vi "Peltier Temperature Test.vi"(8 "error in":errorcluster) -> (0 "error out":errorcluster)   [LabVIEW 2014]
uses:
  CAN Communication/Peltier/Typedefs/Peltier Temperature Sensors.ctl
  CAN Communication/Peltier/Peltier.lvclass
panel:
  in  "Stop":bool
  out "Timeout":i32
  in  "Values":i32(listbox)
  out "Error":errorcluster
  # "Peltier Temperature Test"
  # "This test performs functionality\ntesting on the Peltier Board.\n\nPlease standby while the test is\nin progress..."
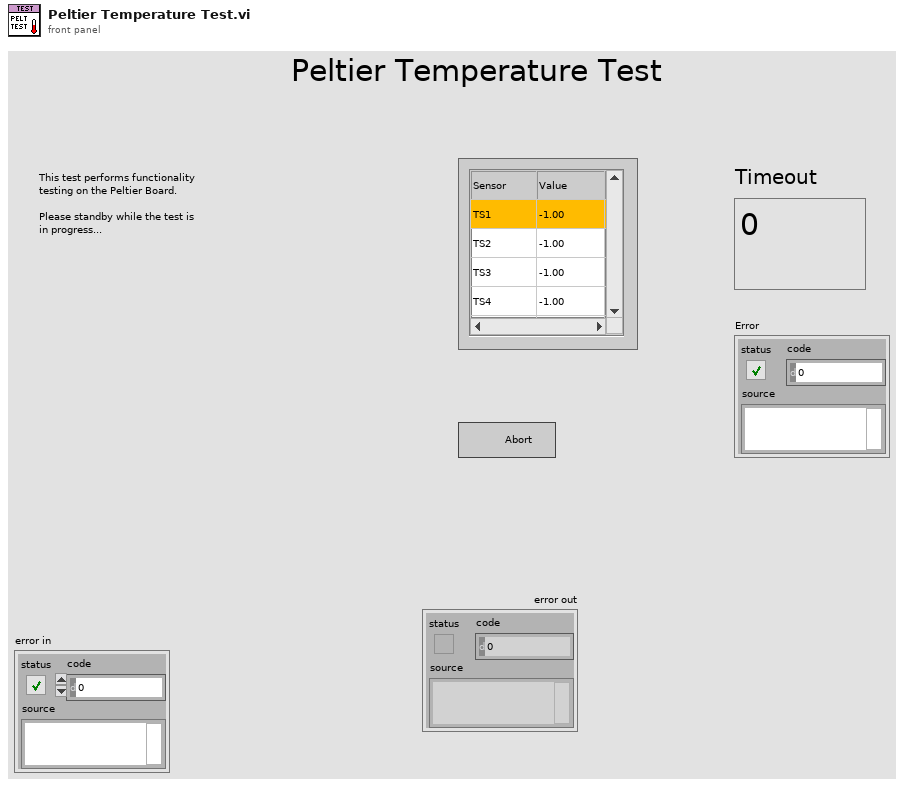
[diagram p1: front panel]
types:
  T1 = typedef "Peltier.lvclass/Peltier Temperature Sensors.ctl" = u16
  T2 = typedef "Peltier.lvclass/Session Handle.ctl" = refnum<data-value>
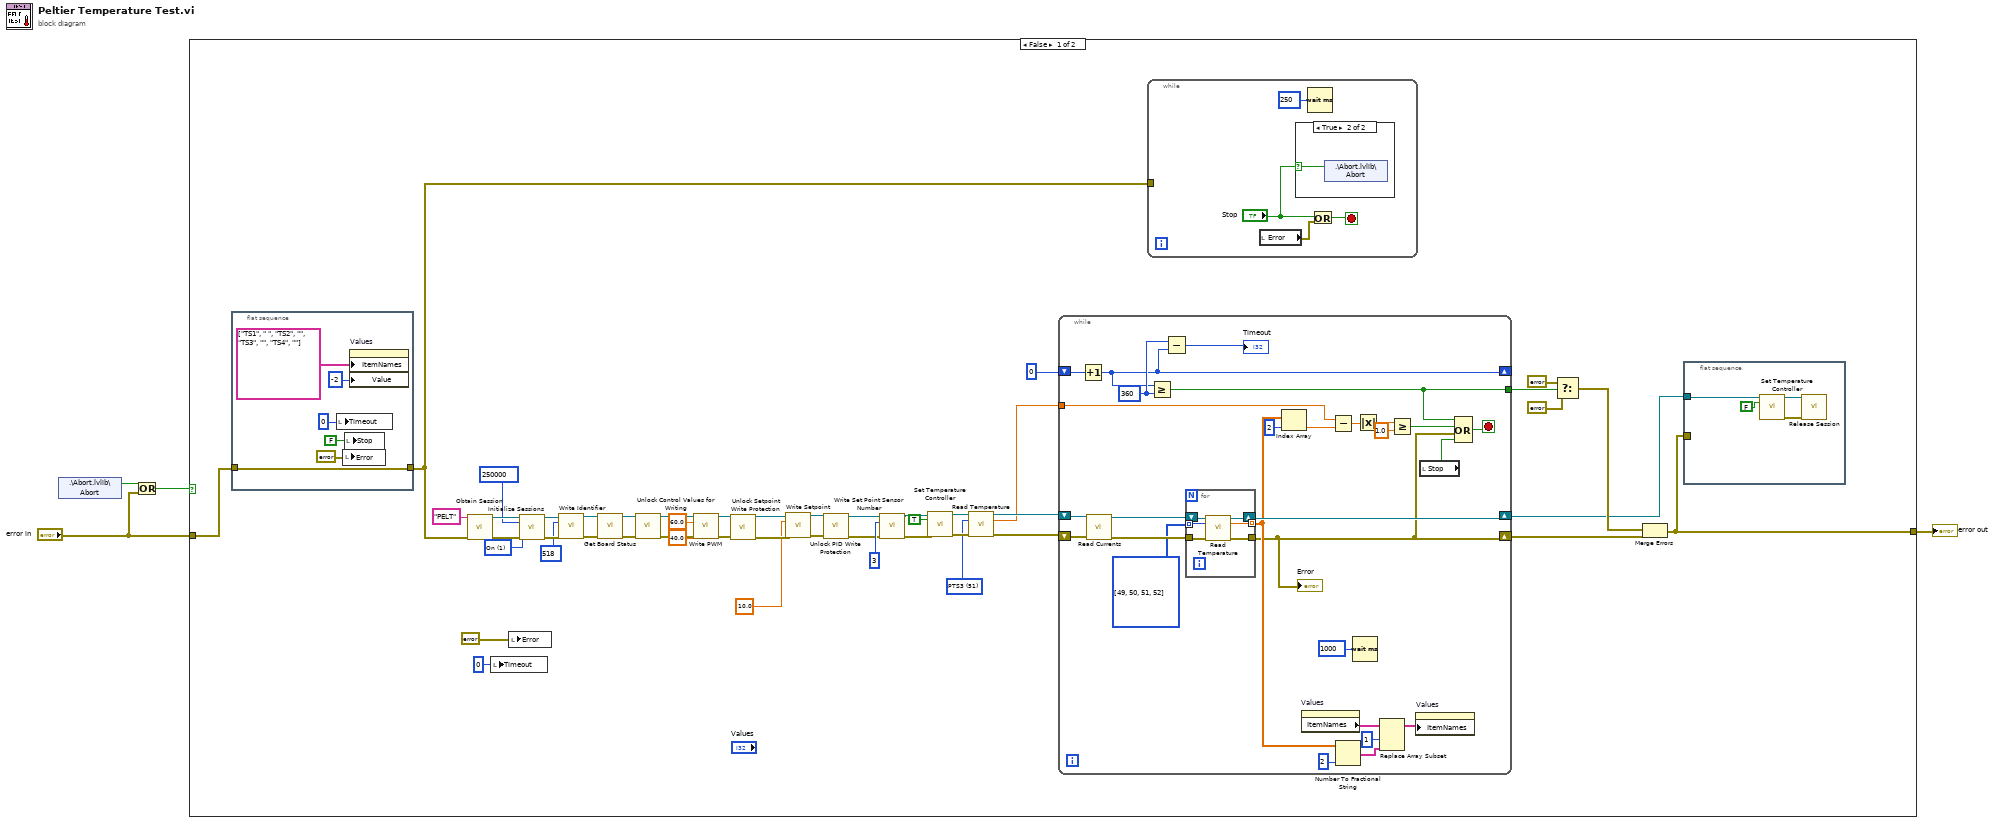
[diagram p0: block diagram]
diagram:
  n1 = shared-variable ".\\Abort.lvlib\\Abort"() -> (w3:bool)  [unwired: 1 in, 1 out]
  n2 = Or(x=w3, y="error in") -> (x .or. y?=w1:bool)
  n3 = case shown="False" w1 {
    tunnel: "error in" -> [w7 w101]
    tunnel: [w5 w101] -> w4
    frame False {
      w21 = T1 51 items=["PTS1"=49, "PTS2"=50, "PTS3"=51, "PTS4"=52, "PTS5"=53, "PTS6"=54] ("Pelt Temp Sensors")
      w47 = u32 1 items=["Off", "On"] ("Termination")
      n4 = flat-sequence {
        tunnel: w7 -> [w56]
        tunnel: [w56] -> w6
        frame #0 {
          n5 = local write "Timeout"(0 ("Timeout")) -> ()
          n6 = local write "Error"(errorcluster {"status"=FALSE, "code"=0, "source"=""} ("Error")) -> ()
          n7 = local write "Stop"(FALSE ("Stop")) -> ()
          n8 = property on="Values" class="MCListbox (strict)"("ItemNames"=string[][] [["TS1", " "], ["TS2", ""], ["TS3", ""], ["TS4", ""]] ("Item Names"), "Value"=-2 ("Values")) -> ()  [unwired: 2 in, 2 out]
        }
      }
      n9 = call "Obtain Session.vi"("Session  Name ()"="PELT", "error in (no error)"=w6) -> ("Session Handle"=w50:T2, "error out"=w49:errorcluster)  [unwired: 12 in]
      n10 = local write "Timeout"(0 ("Timeout")) -> ()
      n11 = local write "Error"(errorcluster {"status"=FALSE, "code"=0, "source"=""} ("Peltier Errors")) -> ()
      n12 = call "Initialize Sessions.vi"("Session Handle"=w50, "Baud Rate"=u32 250000, "Termination"=w47, "error in (no error)"=w49) -> ("Session Handle Out"=w46:T2, "error out"=w45:errorcluster)  [unwired: 10 in]
      n13 = call "Write Identifier.vi"("Session Handle In"=w46, "identifier"=u16 518, "error in (no error)"=w45) -> ("Session Handle Out"=w43:T2, "error out"=w42:errorcluster)  [unwired: 11 in]
      n14 = call "Get Board Status.vi"("Session Handle"=w43, "error in (no error)"=w42) -> ("Session Handle Out"=w13:T2, "error out"=w12:errorcluster)  [unwired: 11 in, 1 out]
      n15 = call "Unlock Control Values for Writing.vi"("Session Handle"=w13, "error in (no error)"=w12) -> ("Session Handle Out"=w33:T2, "error out"=w32:errorcluster)  [unwired: 12 in]
      n16 = call "Write PWM.vi"("Session Handle"=w33, "Max PWM"=60.0, "Min PWM"=40.0, "error in (no error)"=w32) -> ("Session Handle Out"=w29:T2, "error out"=w28:errorcluster)  [unwired: 10 in]
      n17 = call "Unlock Setpoint Write Protection.vi"("Session Handle"=w29, "error in (no error)"=w28) -> ("Session Handle Out"=w37:T2, "error out"=w36:errorcluster)  [unwired: 12 in]
      n18 = call "Write Setpoint.vi"("Session Handle"=w37, "Setpoint"=10.0, "error in (no error)"=w36) -> ("Session Handle Out"=w35:T2, "error out"=w34:errorcluster)  [unwired: 11 in]
      n19 = call "Unlock PID Write Protection.vi"("Session Handle"=w35, "error in (no error)"=w34) -> ("Session Handle Out"=w38:T2, "error out"=w39:errorcluster)  [unwired: 12 in]
      n20 = call "Write Set Point Sensor Number.vi"("Session Handle"=w38, "Sensor Number"=u8 3, "error in (no error)"=w39) -> ("Session Handle Out"=w27:T2, "error out"=w26:errorcluster)  [unwired: 11 in]
      n21 = call "Set Temperature Controller.vi"("Session Handle"=w27, "On?"=TRUE, "error in (no error)"=w26) -> ("Session Handle Out"=w24:T2, "error out"=w25:errorcluster)  [unwired: 11 in]
      n22 = call "Read Temperature.vi"("Session Handle"=w24, "Pelt Temp Sensors"=w21, "error in (no error)"=w25) -> ("Session Handle Out"=w22:T2, "Temperature"=w20:dbl, "error out"=w23:errorcluster)  [unwired: 10 in]
      n23 = while {
        shift-right: [w88] -> w8
        shift-left: w22 -> [w93]
        shift-right: [w74] -> w14
        shift-left: w23 -> [w94]
        tunnel: w20 -> [w79]
        shift-right: [w69] -> _
        shift-left: 0 -> [w72]
        tunnel: [w71] -> w15
        stop <- w73 stop-if-true
        w70 = 360 ("y")
        w90 = T1[] [49, 50, 51, 52] items=["PTS1"=49, "PTS2"=50, "PTS3"=51, "PTS4"=52, "PTS5"=53, "PTS6"=54]
        n24 = Increment(x=w72) -> (x+1=w69:i32)
        n25 = call "Read Currents.vi"("Session Handle"=w93, "error in (no error)"=w94) -> ("Session Handle Out"=w92:T2, "error out"=w91:errorcluster)  [unwired: 10 in, 2 out]
        n26 = Greater Or Equal?(x=w69, y=w70) -> (x >= y?=w71:bool)
        n27 = Subtract(x=w70, y=w69) -> (x-y=→"Timeout":i32)
        n28 = for {
          tunnel: w91 -> [w99]
          shift-right: [w97] -> w88
          shift-left: w92 -> [w100]
          tunnel: [w98] -> w74
          tunnel: [w96] -> w82 mode=indexing
          tunnel: w90 -> [w95] mode=indexing
          n29 = call "Read Temperature.vi"("Session Handle"=w100, "Pelt Temp Sensors"=w95, "error in (no error)"=w99) -> ("Session Handle Out"=w97:T2, "Temperature"=w96:dbl, "error out"=w98:errorcluster)  [unwired: 10 in]
        }
        "Error" <- w74
        n30 = Index Array(array=w82, index=2) -> (element=w80:dbl)
        n31 = property on="Values" class="MCListbox (strict)"() -> ("ItemNames"=w87:string[][])  [unwired: 2 in, 2 out]
        n32 = Subtract(x=w79, y=w80) -> (x-y=w78:dbl)
        n33 = Number To Fractional String(number=w82, precision (6)=i16 2) -> (F-format string=w85:string[])  [unwired: 2 in]
        n34 = Wait (ms)(milliseconds to wait=u32 1000) -> ()  [unwired: 1 out]
        n35 = Absolute Value(x=w78) -> (abs(x)=w77:dbl)
        n36 = Replace Array Subset(array=w87, new element=w85, index (col)=1 ("disabled index (col)")) -> (w84:string[][])  [unwired: 1 in]
        n37 = Greater Or Equal?(x=w77, y=1.0) -> (x >= y?=w75:bool)
        n38 = property on="Values" class="MCListbox (strict)"("ItemNames"=w84) -> ()  [unwired: 2 in, 2 out]
        n39 = local read "Stop"() -> (w67:bool)
        n40 = Compound Arithmetic op=OR(w71, w75, w74, w67) -> (w73:bool)
      }
      n41 = while {
        tunnel: w6 -> [_]
        stop <- w58 stop-if-true
        n42 = local read "Error"() -> (w59:errorcluster)
        n43 = case shown="True" "Stop" {
          selector: "Stop" -> [_ w62]
          frame False {
          }
          frame True {
            n44 = shared-variable ".\\Abort.lvlib\\Abort"(w62) -> ()  [unwired: 1 in, 1 out]
          }
        }
        n45 = Wait (ms)(milliseconds to wait=u32 250) -> ()  [unwired: 1 out]
        n46 = Or(x="Stop", y=w59) -> (x .or. y?=w58:bool)
      }
      n47 = Select(t=errorcluster {"status"=TRUE, "code"=9001, "source"="Timeout Error. Peltier Controller Failed to Reach Setpoint."} ("error out"), s=w15, f=errorcluster {"status"=FALSE, "code"=0, "source"=""} ("error out")) -> (s? t:f=w16:errorcluster)
      n48 = Merge Errors(w16, w14) -> (w5:errorcluster)
      n49 = flat-sequence {
        tunnel: w5 -> [_]
        tunnel: w8 -> [w65]
        frame #0 {
          n50 = call "Set Temperature Controller.vi"("Session Handle"=w65, "On?"=FALSE) -> ("Session Handle Out"=w63:T2, "error out"=w64:errorcluster)  [unwired: 12 in]
          n51 = call "Release Session.vi"("Session Handle"=w63, "error in (no error)"=w64) -> ()  [unwired: 13 in, 1 out]
        }
      }
    }
    frame True {
    }
  }
  "error out" <- w4
